vi "Read TDMS Wave 1D.vi"(8 "error in (no error)":errorcluster, 10 "channel name(s) in":string, 11 "path":path) -> (0 "error out":errorcluster, 2 "data":dbl[](array[numeric]), 3 "file path out":path)   [LabVIEW 2016, in "Data.TDMS.lvclass"]
uses:
  Data.TDMS.lvclass
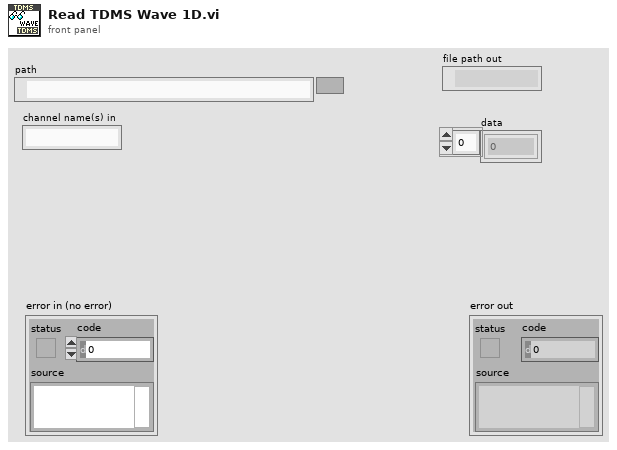
[diagram p1: front panel]
types:
  T1 = enum16{"open", "open or create", "create or replace", "create", "open (read-only)"}
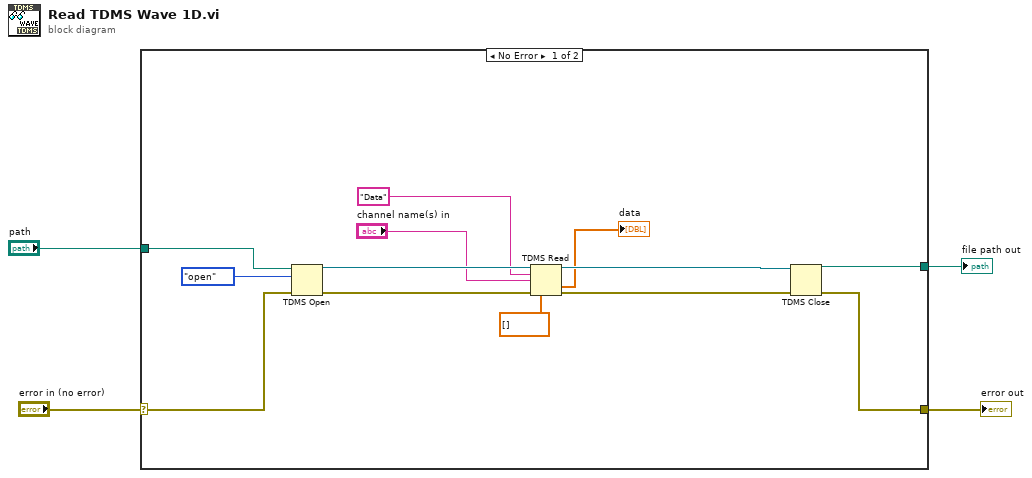
[diagram p0: block diagram]
diagram:
  n1 = case shown="No Error" "error in (no error)" {
    selector: "error in (no error)" -> [w6 w18]
    tunnel: [w16 w18] -> w3
    tunnel: "path" -> [w13 _]
    tunnel: [w5 _] -> w1
    frame No Error {
      n2 = TDMS Open(8:w6, 10:T1."open" ("operation (0:open)"), 11:w13) -> (0:w11:errorcluster, 3:w10:refnum<k34>)  [unwired: 4 in]
      n3 = TDMS Read(0:w10, 5:"Data" ("group name"), 7:"channel name(s) in", 11:w11, 12:dbl[] [] ("array type (2D Dbl)")) -> (4:w15:refnum<k34>, 10:→"data":dbl[], 15:w14:errorcluster)  [unwired: 3 in, 3 out]
      n4 = TDMS Close(8:w14, 11:w15) -> (0:w16:errorcluster, 3:w5:path)
    }
    frame Error {
    }
  }
  "error out" <- w3
  "file path out" <- w1
